vi "TCP Read.vi"(3 "error in (no error)":errorcluster, 4 "Data to Write":T1={"Array of Motor Speeds"=[0.0, 0.0, 0.0, 0.0]}, 5 "connection ID":refnum<k5>) -> (0 "error out":errorcluster, 1 "Data read":cluster{"Array of Motor Speeds":dbl[]}, 2 "connection ID out":refnum<k5>)   [LabVIEW 2018]
uses:
  controls/TCP Write select.ctl
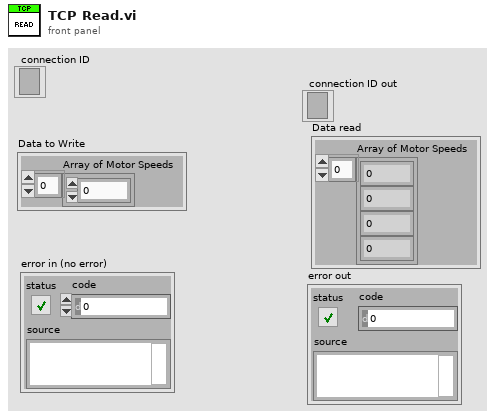
[diagram p1: front panel]
types:
  T1 = typedef "TCP Write select.ctl" = cluster{"Array of Motor Speeds":dbl[]}
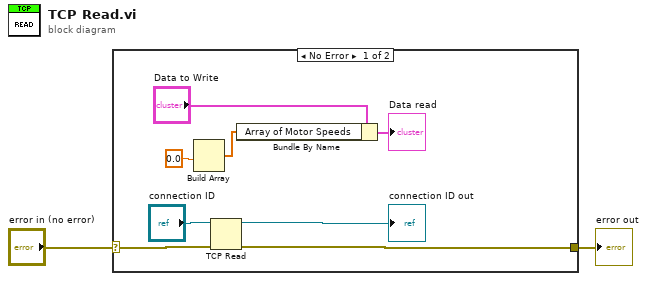
[diagram p0: block diagram]
diagram:
  n1 = case shown="No Error" "error in (no error)" {
    selector: "error in (no error)" -> [w9 w11]
    tunnel: [w8 w11] -> w1
    frame No Error {
      n2 = Build Array(0.0 ("element")) -> (w3:dbl[])  [unwired: 3 in]
      n3 = TCP Read(connection ID="connection ID", error in (no error)=w9) -> (connection ID out=→"connection ID out":refnum<k5>, error out=w8:errorcluster)  [unwired: 3 in, 1 out]
      n4 = Bundle By Name(cluster="Data to Write", "Array of Motor Speeds"=w3) -> (→"Data read":T1)
    }
    frame Error {
      # "if error, do nothing"
    }
  }
  "error out" <- w1
